vi "SetVIWindowTransparency.vi"(7 "VIPath":path, 10 "ErrorIn":errorcluster) -> (2 "ErrorOut":errorcluster)   [LabVIEW 2018]
doc: "Sets the transparency property of the VI specified by VIPath (hides the VI).\n\nUse this before opening another modal window to make a calling VI invisible.\n\nAlso see RestoreVIWindowTransparency.vi."
panel:
  # "Copyright © 2019 Epimedia, Inc. All Rights Reserved.\n\nThe Epimedia Application Library is Copyright © 2009-2017 Epimedia, Inc. \nAll Rights Reserved. Used under license."
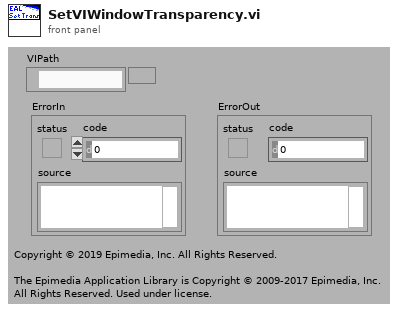
[diagram p1: front panel]
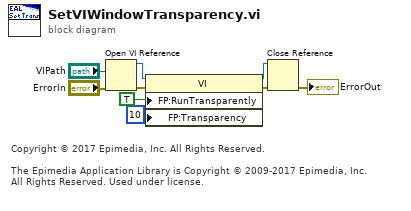
[diagram p0: block diagram]
diagram:
  # "Copyright © 2017 Epimedia, Inc. All Rights Reserved.\n\nThe Epimedia Application Library is Copyright © 2009-2017 Epimedia, Inc. \nAll Rights Reserved. Used under license."
  n1 = Open VI Reference(vi path="VIPath", error in (no error)="ErrorIn") -> (vi reference=w9:refnum<vi>, error out=w8:errorcluster)  [unwired: 4 out]
  n2 = property class="VI"(reference=w9, error in=w8, "FP:RunTransparently"=TRUE ("Front Panel Window:Run VI Transparently"), "FP:Transparency"=u8 10 ("Front Panel Window:Transparency")) -> (reference out=w3:refnum<vi>, error out=w5:errorcluster)
  n3 = Close Reference(reference=w3, error in (no error)=w5) -> (error out=→"ErrorOut":errorcluster)
